vi "Open Call By VIs.vi"(10 "Call By Refs":T1, 11 "App Path":path) -> (2 "error out":errorcluster, 3 "Call By Refs OUT":T1)   [LabVIEW 2019]
uses:
  Type Defs and Controls/Call By Refs.ctl
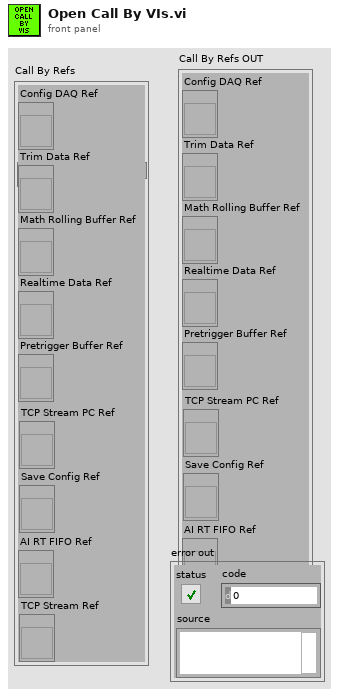
[diagram p1: front panel]
types:
  T1 = typedef "Call By Refs.ctl" = cluster{"Config DAQ Ref":refnum<vi>, "Trim Data Ref":refnum<vi>, "Math Rolling Buffer Ref":refnum<vi>, "Realtime Data Ref":refnum<vi>, "Pretrigger Buffer Ref":refnum<vi>, "TCP Stream PC Ref":refnum<vi>, "Save Config Ref":refnum<vi>, "AI RT FIFO Ref":refnum<vi>, "TCP Stream Ref":refnum<vi>}
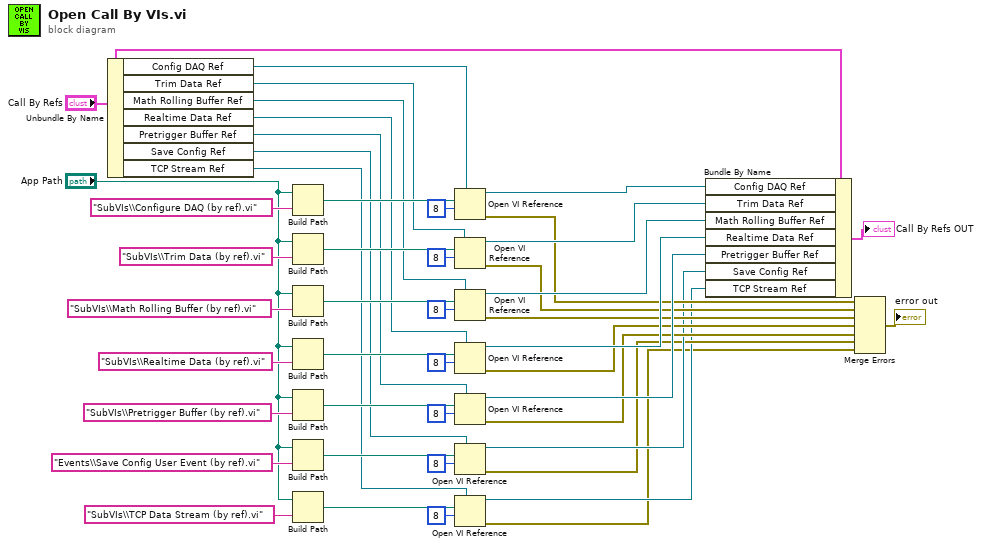
[diagram p0: block diagram]
diagram:
  n1 = Unbundle By Name("Call By Refs") -> ("Config DAQ Ref"=w43:refnum<vi>, "Trim Data Ref"=w30:refnum<vi>, "Math Rolling Buffer Ref"=w29:refnum<vi>, "Realtime Data Ref"=w28:refnum<vi>, "Pretrigger Buffer Ref"=w27:refnum<vi>, "Save Config Ref"=w9:refnum<vi>, "TCP Stream Ref"=w4:refnum<vi>)
  n2 = Build Path(base path="App Path", name or relative path="SubVIs\\Configure DAQ (by ref).vi") -> (appended path=w45:path)
  n3 = Build Path(base path="App Path", name or relative path="SubVIs\\Trim Data (by ref).vi") -> (appended path=w41:path)
  n4 = Build Path(base path="App Path", name or relative path="SubVIs\\Math Rolling Buffer (by ref).vi") -> (appended path=w38:path)
  n5 = Build Path(base path="App Path", name or relative path="SubVIs\\Realtime Data (by ref).vi") -> (appended path=w35:path)
  n6 = Build Path(base path="App Path", name or relative path="SubVIs\\Pretrigger Buffer (by ref).vi") -> (appended path=w32:path)
  n7 = Build Path(base path="App Path", name or relative path="Events\\Save Config User Event (by ref).vi") -> (appended path=w12:path)
  n8 = Build Path(base path="App Path", name or relative path="SubVIs\\TCP Data Stream (by ref).vi") -> (appended path=w6:path)
  n9 = Open VI Reference(type specifier VI Refnum (for type only)=w43, vi path=w45, options=8) -> (vi reference=w25:refnum<vi>, error out=w19:errorcluster)  [unwired: 3 in]
  n10 = Open VI Reference(type specifier VI Refnum (for type only)=w30, vi path=w41, options=8) -> (vi reference=w24:refnum<vi>, error out=w18:errorcluster)  [unwired: 3 in]
  n11 = Open VI Reference(type specifier VI Refnum (for type only)=w29, vi path=w38, options=8) -> (vi reference=w23:refnum<vi>, error out=w17:errorcluster)  [unwired: 3 in]
  n12 = Open VI Reference(type specifier VI Refnum (for type only)=w28, vi path=w35, options=8) -> (vi reference=w22:refnum<vi>, error out=w16:errorcluster)  [unwired: 3 in]
  n13 = Open VI Reference(type specifier VI Refnum (for type only)=w27, vi path=w32, options=8) -> (vi reference=w21:refnum<vi>, error out=w15:errorcluster)  [unwired: 3 in]
  n14 = Open VI Reference(type specifier VI Refnum (for type only)=w9, vi path=w12, options=8) -> (vi reference=w10:refnum<vi>, error out=w8:errorcluster)  [unwired: 3 in]
  n15 = Open VI Reference(type specifier VI Refnum (for type only)=w4, vi path=w6, options=8) -> (vi reference=w3:refnum<vi>, error out=w2:errorcluster)  [unwired: 3 in]
  n16 = Bundle By Name(cluster="Call By Refs", "Config DAQ Ref"=w25, "Trim Data Ref"=w24, "Math Rolling Buffer Ref"=w23, "Realtime Data Ref"=w22, "Pretrigger Buffer Ref"=w21, "Save Config Ref"=w10, "TCP Stream Ref"=w3) -> (→"Call By Refs OUT":T1)
  n17 = Merge Errors(w19, w18, w17, w16, w15, w8, w2) -> (→"error out":errorcluster)
